vi "CompPtGUI.vi"(5 "error in (no error)":errorcluster) -> (16 "output cluster":T1, 19 "error out":errorcluster)   [LabVIEW 2018]
panel:
  in  "Compression Pt.":enum16{".1", ".3", "1", "3"}(ring)=enum."1"
  in  "stop":bool
  in  "OK Button":bool
  in  "CW Frequency":dbl=2000000000.0 format="%_3g"
  in  "Format":string(combo)="MLOGarithmic"
  in  "Average?":bool=TRUE
  in  "Avg. Factor":i32=20
  in  "Stop Power":i32=10
  in  "Start Power":i32=-20
  # "Compression PT Measurement Parameters"
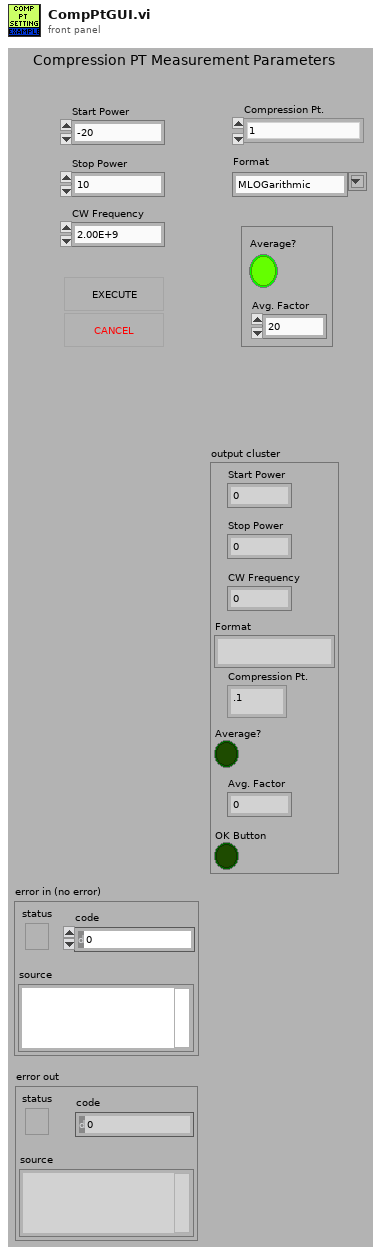
[diagram p1: front panel]
types:
  T1 = cluster{"Start Power":i32, "Stop Power":i32, "CW Frequency":dbl, "Format":string, "Compression Pt.":enum16{".1", ".3", "1", "3"}, "Average?":bool, "Avg. Factor":i32, "OK Button":bool}
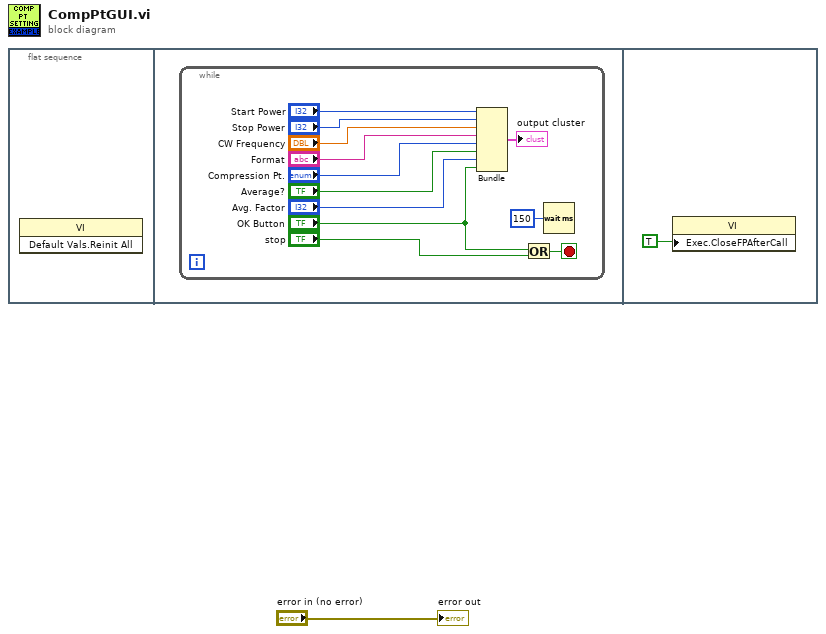
[diagram p0: block diagram]
diagram:
  n1 = flat-sequence {
    frame #0 {
      n2 = invoke class="VI" method="Default Vals.Reinit All"() -> ()  [unwired: 3 in, 3 out]
    }
    frame #1 {
      n3 = while {
        stop <- w6 stop-if-true
        n4 = Bundle("Start Power"="Start Power", "Stop Power"="Stop Power", "CW Frequency"="CW Frequency", "Format"="Format", "Compression Pt."="Compression Pt.", "Average?"="Average?", "Avg. Factor"="Avg. Factor", "OK Button"="OK Button") -> (→"output cluster":T1)  [unwired: 1 in]
        n5 = Or(x="OK Button", y="stop") -> (x .or. y?=w6:bool)
        n6 = Wait (ms)(milliseconds to wait=u32 150) -> ()  [unwired: 1 out]
      }
    }
    frame #2 {
      n7 = property class="VI"("Exec.CloseFPAfterCall"=TRUE ("Execution:Close After Call")) -> ()  [unwired: 2 in, 2 out]
    }
  }
  "error out" <- "error in (no error)"
